vi "Handle Line Control Change.vi"(8 "error in (no error)":errorcluster, 9 "Interlock Chain":refnum<class "Interlock Chain.lvclass">, 10 "Requested Bitfield":u16, 11 "Storage Line in":refnum<class "Storage Line.lvclass">) -> (0 "error out":errorcluster, 3 "Storage Line out":refnum<class "Storage Line.lvclass">)   [LabVIEW 2015, in "cRIO-Carbondioxide.lvlib" / "CO2-Actor.lvlib" / "Storage Line.lvclass"]
uses:
  Storage Line.lvclass
  Interlocks/Interlock Chain/Interlock Chain.lvclass
  Storage Line.lvclass/Storage Line.ctl
  <vilib>/ActorFramework/Actor/Actor.lvclass/Actor.ctl
  <vilib>/ActorFramework/Message Enqueuer/Message Enqueuer.lvclass/Message Enqueuer.ctl
  Storage Line Messages/Set Line Msg/Set Line Msg.lvclass/Set Line Msg.ctl
  CO2 Actor Messages/Wait Msg/Wait Msg.lvclass/Wait Msg.ctl
  <vilib>/ActorFramework/Actor/Read Self Enqueuer.vi
  <vilib>/ActorFramework/Message Enqueuer/Enqueue.vi
  <vilib>/ActorFramework/Message Enqueuer/Init from Existing Queue.vi
  <vilib>/ActorFramework/Message Priority Queue/Priority Enqueue.vi
  <vilib>/ActorFramework/Actor/Actor.lvclass
  <vilib>/ActorFramework/Message Enqueuer/Message Enqueuer.lvclass
  Storage Line Messages/Set Line Msg/Set Line Msg.lvclass
  CO2 Actor Messages/Wait Msg/Wait Msg.lvclass
  CO2 Actor/CO2 Actor.lvclass
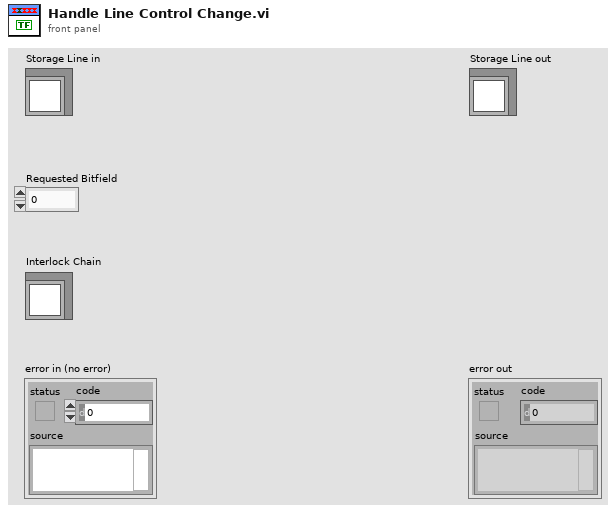
[diagram p1: front panel]
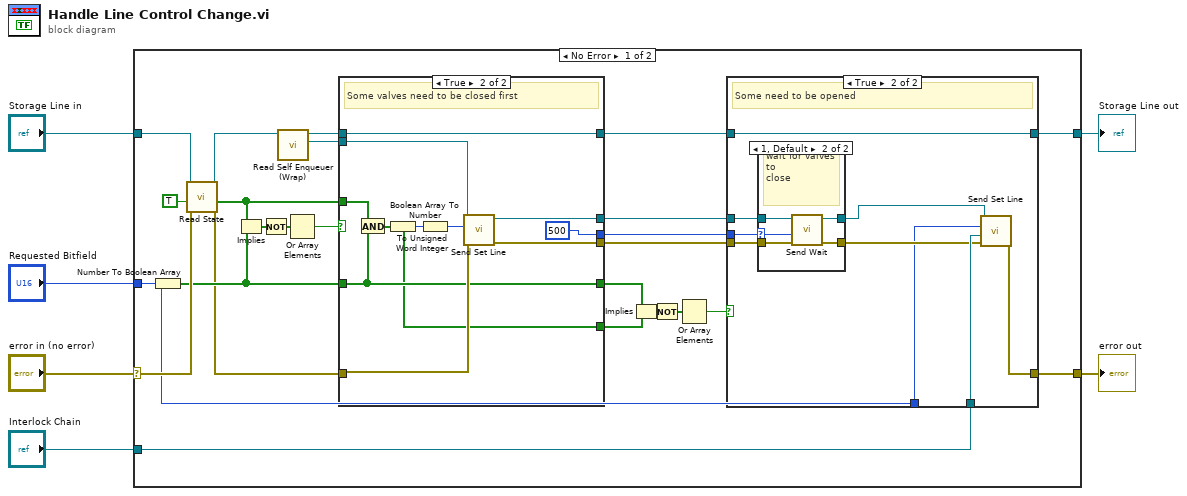
[diagram p0: block diagram]
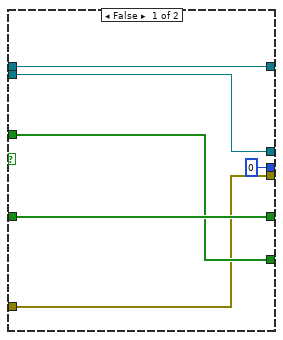
[diagram p4: hidden frame]
diagram:
  n1 = case shown="No Error" "error in (no error)" {
    selector: "error in (no error)" -> [w31 w68]
    tunnel: [w9 w68] -> w5
    tunnel: [w11 w67] -> w3
    tunnel: "Storage Line in" -> [w30 w67]
    tunnel: "Requested Bitfield" -> [w8 _]
    tunnel: "Interlock Chain" -> [w7 _]
    frame No Error {
      n2 = Number To Boolean Array(number=w8) -> (Boolean array=w26:bool[])
      n3 = call "Read State.vi"("error in (no error)"=w31, "Return Boolean Array? (F)"=TRUE, "Storage Line in"=w30) -> ("error out"=w22:errorcluster, "Boolean array"=w27:bool[], "Storage Line out"=w25:refnum<class "Storage Line.lvclass">)  [unwired: 4 in, 2 out]
      n4 = Implies(1:w26, 2:w27) -> (0:w20:bool[])
      n5 = Not(x=w20) -> (.not. x?=w19:bool[])
      n6 = call "Read Self Enqueuer (Wrap).vi"("CO2 Actor in"=w25) -> ("Actor Framework:Message Enqueuer"=w23:refnum<class "Message Enqueuer.lvclass">, "CO2 Actor out"=w24:refnum<class "Storage Line.lvclass">)  [unwired: 9 in]
      n7 = Or Array Elements(Boolean array=w19) -> (logical OR=w28:bool)
      n8 = case shown="True" w28 {
        tunnel: [w55 w66] -> w15
        tunnel: w24 -> [w55 w66]
        tunnel: w27 -> [w53 w61]
        tunnel: w26 -> [w54 w60]
        tunnel: w23 -> [w52 w62]
        tunnel: w22 -> [w51 w63]
        tunnel: [w54 w60] -> w10
        tunnel: [w53 w59] -> w21
        tunnel: [w51 w58] -> w13
        tunnel: [u32 0 ("milliseconds to wait") u32 500 ("milliseconds to wait")] -> w12
        tunnel: [w52 w56] -> w14
        frame False {
        }
        frame True {
          # "Some valves need to be closed first"
          n9 = And(x=w61, y=w60) -> (x .and. y?=w59:bool[])
          n10 = Boolean Array To Number(Boolean array=w59) -> (number=w65:u32)
          n11 = To Unsigned Word Integer(number=w65) -> (unsigned 16bit integer=w64:u16)
          n12 = call "Send Set Line.vi"("error in (no error)"=w63, "Bit Field"=w64, "Message Enqueuer"=w62) -> ("error out"=w58:errorcluster, "Message Enqueuer out"=w56:refnum<class "Message Enqueuer.lvclass">)  [unwired: 7 in]
        }
      }
      n13 = Implies(1:w21, 2:w10) -> (0:w18:bool[])
      n14 = Not(x=w18) -> (.not. x?=w17:bool[])
      n15 = Or Array Elements(Boolean array=w17) -> (logical OR=w16:bool)
      n16 = case shown="True" w16 {
        tunnel: w15 -> [w33 w35]
        tunnel: w14 -> [_ w42]
        tunnel: w13 -> [w32 w41]
        tunnel: w12 -> [_ w40]
        tunnel: [w33 w35] -> w11
        tunnel: w8 -> [_ w34]
        tunnel: [w32 w38] -> w9
        tunnel: w7 -> [_ w37]
        frame False {
        }
        frame True {
          # "Some need to be opened"
          n17 = case shown="1, Default" w40 {
            selector: w40 -> [_ w46]
            tunnel: w42 -> [w44 w49]
            tunnel: w41 -> [w43 w48]
            tunnel: [w43 w47] -> w36
            tunnel: [w44 w45] -> w39
            frame 0 {
            }
            frame 1, Default {
              # "wait for valves to\nclose"
              n18 = call "Send Wait.vi"("error in (no error)"=w48, "milliseconds to wait"=w46, "Message Enqueuer"=w49) -> ("error out"=w47:errorcluster, "Message Enqueuer out"=w45:refnum<class "Message Enqueuer.lvclass">)  [unwired: 7 in]
            }
          }
          n19 = call "Send Set Line.vi"("error in (no error)"=w36, "Interlock Chain"=w37, "Bit Field"=w34, "Message Enqueuer"=w39) -> ("error out"=w38:errorcluster)  [unwired: 6 in, 1 out]
        }
      }
    }
    frame Error {
    }
  }
  "error out" <- w5
  "Storage Line out" <- w3
